vi "File to PG.vi"(6 "Numeric":i32, 8 "error in (no error)":errorcluster, 10 "Path":path, 11 "Conversion.lvclass":refnum<class "Conversion.lvclass">) -> (0 "error out":errorcluster, 2 "Not Equal?":bool, 3 "Conversion.lvclass out":refnum<class "Conversion.lvclass">)   [LabVIEW 2016, in "Conversion.lvclass"]
uses:
  Conversion.lvclass
  Conversion.lvclass/Conversion.ctl
  Data/Typedefs/File Type--enum.ctl
  Data/Typedefs/Operation--enum.ctl
  Data/Data.lvclass
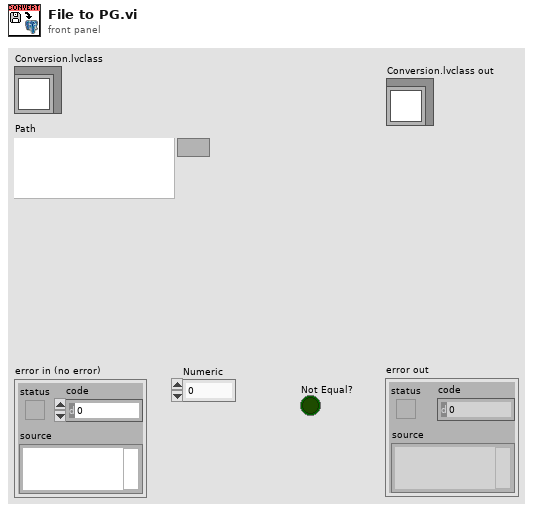
[diagram p1: front panel]
types:
  T1 = typedef "Data.lvclass/Operation--enum.ctl" = enum16{"Read", "Write", "Write + Append"}
  T2 = typedef "Data.lvclass/Dictionary--cluster.ctl" = cluster{"key":string, "value":variant}
  T3 = typedef "Data.lvclass/File Type--enum.ctl" = enum16{"DAT", "ITX", "TDMS", "VI", "PGSQL"}
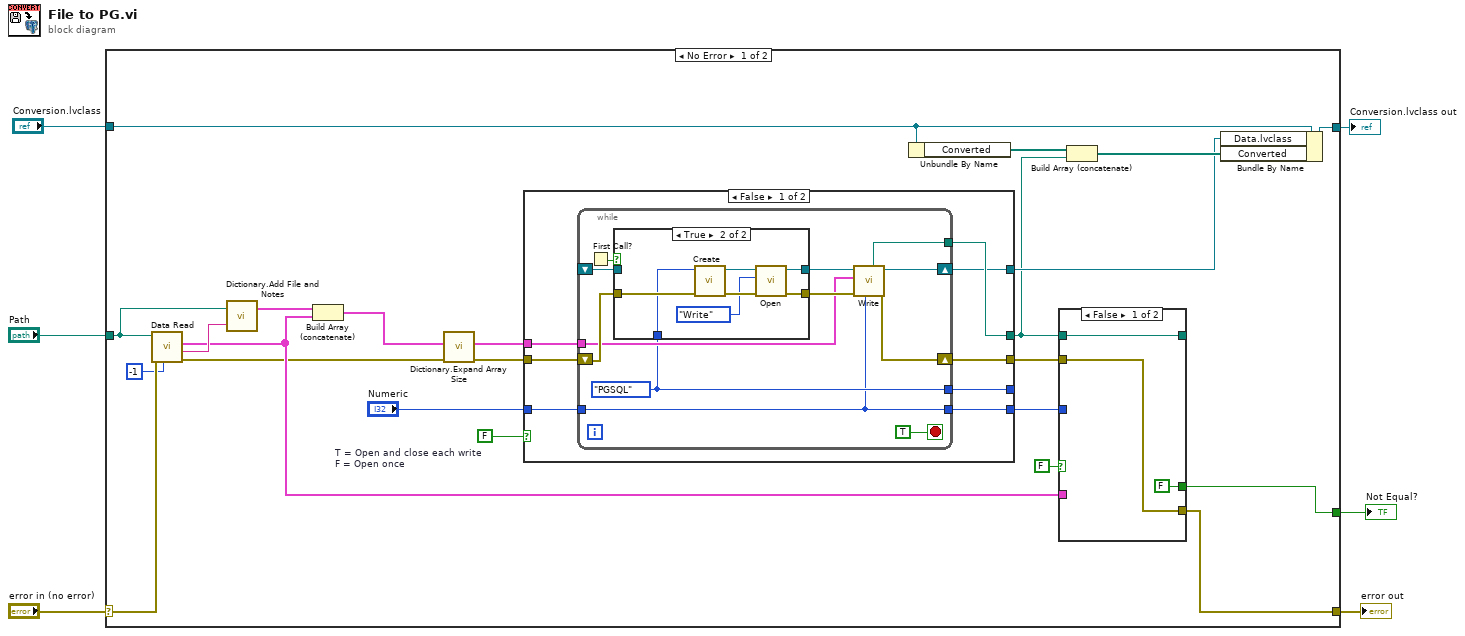
[diagram p0: block diagram]
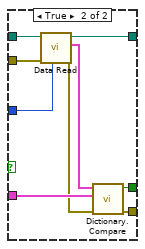
[diagram p2: hidden frame]
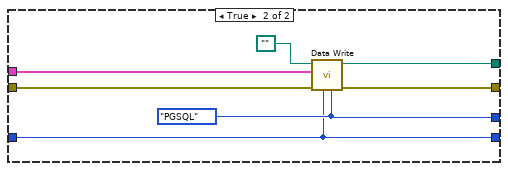
[diagram p4: hidden frame]
diagram:
  n1 = case shown="No Error" "error in (no error)" {
    selector: "error in (no error)" -> [w29 w79]
    tunnel: [w10 w79] -> w5
    tunnel: "Path" -> [w20 _]
    tunnel: [w11 _] -> w3
    tunnel: "Conversion.lvclass" -> [w14 w78]
    tunnel: [w8 w78] -> w1
    frame No Error {
      w27 = FALSE  # T = Open and close each write F = Open once
      n2 = call "Data Read.vi"("Append Index"=-1, "error in (no error)"=w29, "path"=w20) -> ("error out"=w19:errorcluster, "Notes"=w24:string, "Data (Dictionary)"=w21:T2[])  [unwired: 5 in, 1 out]
      n3 = call "Dictionary.Add File and Notes.vi"("Notes"=w24, "Path"=w20) -> ("Dictionary"=w23:T2[])  [unwired: 1 in]
      n4 = Build Array (concatenate)(w23, w21) -> (w22:T2[])
      n5 = call "Dictionary.Expand Array Size.vi"("error in (no error)"=w19, "Data (Dictionary)"=w22) -> ("error out"=w25:errorcluster, "Data (Dictionary)"=w26:T2[])  [unwired: 8 in]
      n6 = case shown="False" w27 {
        tunnel: [w45 w77] -> w12
        tunnel: [w48 w76] -> w28
        tunnel: w26 -> [w47 w75]
        tunnel: w25 -> [w49 w74]
        tunnel: [w46 w73] -> _
        tunnel: [w44 _] -> w13
        tunnel: "Numeric" -> [w43 w71]
        tunnel: [w42 w71] -> w9
        frame False {
          n7 = while {
            tunnel: w47 -> [w57]
            tunnel: [w53] -> w46
            shift-right: [w58] -> w48
            shift-left: w49 -> [w59]
            shift-right: [w56] -> w44
            shift-left: _ -> [w54]
            tunnel: [w51] -> w45
            tunnel: w43 -> [w50]
            tunnel: [w50] -> w42
            stop <- TRUE stop-if-true
            w53 = File_Type--enum."PGSQL" ("File Type")
            n8 = First Call?() -> (First Call?: T/F=w55:bool)
            n9 = case shown="True" w55 {
              tunnel: [w62 w70] -> w61
              tunnel: [w63 w69] -> w60
              tunnel: w59 -> [w62 w66]
              tunnel: w53 -> [_ w65]
              tunnel: w54 -> [w63 _]
              frame False {
              }
              frame True {
                n10 = call "Create.vi"("error in (no error)"=w66, "File Type"=w65) -> ("error out"=w67:errorcluster, "Data out"=w68:refnum<class "Data.lvclass">)  [unwired: 8 in]
                n11 = call-dynamic "Open.vi"("error in (no error)"=w67, "Operation"=Operation--enum."Write", "Data in"=w68) -> ("error out"=w70:errorcluster, "Data out"=w69:refnum<class "Data.lvclass">)  [unwired: 7 in]
              }
            }
            n12 = call-dynamic "Write.vi"("Append Index"=w50, "error in (no error)"=w61, "Data (Dictionary)"=w57, "Data in"=w60) -> ("error out"=w58:errorcluster, "Data out"=w56:refnum<class "Data.lvclass">, "Path out"=w51:path)  [unwired: 5 in]
          }
        }
        frame True {
          w73 = File_Type--enum."PGSQL" ("File Type")
          n13 = call "Data Write.vi"("File Type"=w73, "Append Index"=w71, "error in (no error)"=w74, "Data (Dictionary)"=w75, "path"=path "") -> ("error out"=w76:errorcluster, "path out"=w77:path)  [unwired: 5 in]
        }
      }
      n14 = Unbundle By Name(w14) -> ("Converted"=w16:path[])
      n15 = case shown="False" FALSE {
        tunnel: w28 -> [w31 w41]
        tunnel: [w32 w40] -> _
        tunnel: w21 -> [_ w39]
        tunnel: w12 -> [w32 w38]
        tunnel: [FALSE ("Not Equal?") w35] -> w11
        tunnel: [w31 w34] -> w10
        tunnel: w9 -> [_ w33]
        frame False {
        }
        frame True {
          n16 = call "Data Read.vi"("Append Index"=w33, "error in (no error)"=w41, "path"=w38) -> ("error out"=w36:errorcluster, "Data (Dictionary)"=w37:T2[], "path out"=w40:path)  [unwired: 5 in, 1 out]
          n17 = call "Dictionary.Compare.vi"("error in (no error)"=w36, "Original Data (Dictionary)"=w39, "Converted Data (Dictionary)"=w37) -> ("error out"=w34:errorcluster, "Not Equal?"=w35:bool)  [unwired: 7 in]
        }
      }
      n18 = Build Array (concatenate)(w16, w12) -> (w15:path[])
      n19 = Bundle By Name(cluster=w14, "Data.lvclass"=w13, "Converted"=w15) -> (w8:refnum<class "Conversion.lvclass">)
    }
    frame Error {
    }
  }
  "error out" <- w5
  "Not Equal?" <- w3
  "Conversion.lvclass out" <- w1
